vi "SVN Read Method.vi"(6 "Which Method Type":T1, 8 "error in (no error)":errorcluster, 9 "Method version":i32, 10 "Method Name":string) -> (0 "error out":errorcluster, 1 "Valid method":bool, 3 "Method text":string)   [LabVIEW 2012]
uses:
  Which method type.ctl
  ReadWrite.ctl
  Folders.ctl
  Design Server.lvlib
panel:
  out "standard error":string
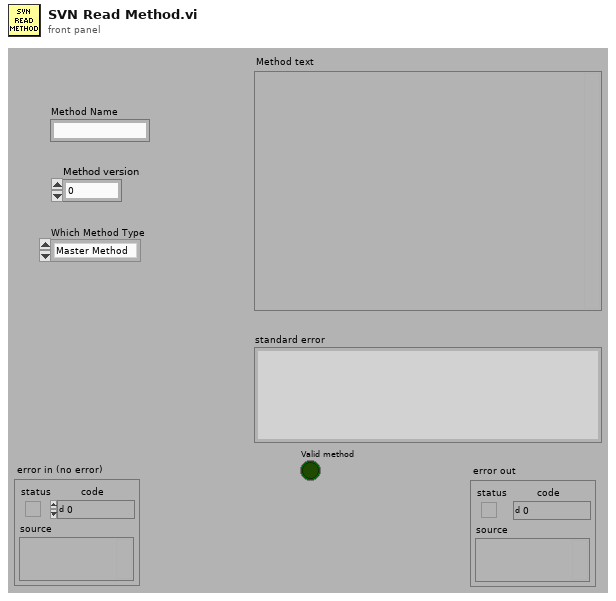
[diagram p1: front panel]
types:
  T1 = typedef "Which method type.ctl" = enum16{"Master Method", "Method"}
  T2 = typedef "Design Server.lvlib/Folders.ctl" = enum16{"MathcadMethods", "RequestedDesigns", "CompletedDesigns", "MathcadCode", "CollabnetSVN.exe"}
  T3 = typedef "ReadWrite.ctl" = enum16{"Read", "Write"}
  T4 = typedef "SVN.ctl" = cluster{"Mathcad Code Repository":string, "Username":string, "Password":string, "Method file names (w extension)":string}
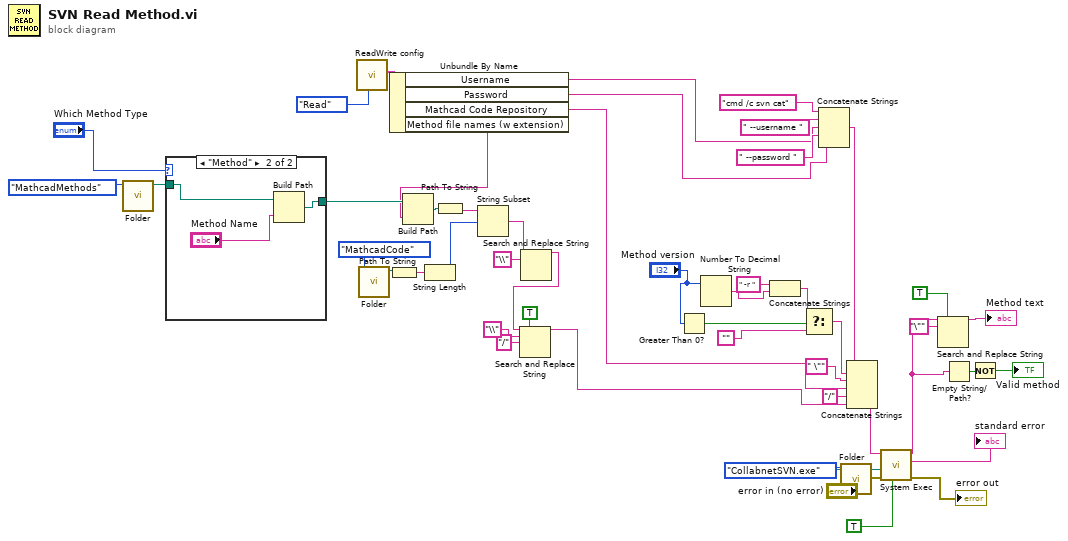
[diagram p0: block diagram]
diagram:
  n1 = call "Folder.vi"("Folders"=Folders."MathcadMethods") -> ("FolderPath"=w22:path)  [unwired: 8 in, 2 out]
  n2 = case shown="\"Method\"" "Which Method Type" {
    tunnel: w22 -> [w50 w53]
    tunnel: [w50 w52] -> w19
    frame "Master Method", Default {
    }
    frame "Method" {
      n3 = Build Path(base path=w53, name or relative path="Method Name") -> (appended path=w52:path)
    }
  }
  n4 = call "ReadWrite config.vi"("Config"=ReadWrite."Read") -> ("SVN"=w37:T4)  [unwired: 7 in, 3 out]
  n5 = call "Folder.vi"("Folders"=Folders."MathcadCode") -> ("FolderPath"=w25:path)  [unwired: 8 in, 2 out]
  n6 = Path To String(path=w25) -> (string=w26:string)
  n7 = Unbundle By Name(w37) -> ("Username"=w34:string, "Password"=w36:string, "Mathcad Code Repository"=w29:string, "Method file names (w extension)"=w1:string)
  n8 = Build Path(base path=w19, name or relative path=w1) -> (appended path=w20:path)
  n9 = String Length(string=w26) -> (length=w21:i32)
  n10 = Path To String(path=w20) -> (string=w17:string)
  n11 = String Subset(string=w17, offset (0)=w21) -> (substring=w18:string)  [unwired: 1 in]
  n12 = Search and Replace String(input string=w18, search string="\\") -> (result string=w12:string)  [unwired: 6 in, 3 out]
  n13 = Search and Replace String(replace all?=TRUE ("replace all? (F)"), input string=w12, search string="\\", replace string="/" ("replace string (\"\")")) -> (result string=w11:string)  [unwired: 4 in, 3 out]
  n14 = Greater Than 0?(x="Method version") -> (x > 0?=w44:bool)
  n15 = Number To Decimal String(number="Method version") -> (decimal integer string=w40:string)  [unwired: 1 in]
  n16 = Concatenate Strings(" -r " ("string"), w40) -> (w42:string)
  n17 = Select(t=w42, s=w44, f="") -> (s? t:f=w39:string)
  n18 = Concatenate Strings("cmd /c svn cat" ("command"), " --username " ("string"), w34, " --password " ("string"), w36) -> (w30:string)
  n19 = call "Folder.vi"("Folders"=Folders."CollabnetSVN.exe") -> ("FolderPath"=w27:path)  [unwired: 8 in, 2 out]
  n20 = Concatenate Strings(w30, w39, " \"" ("string"), w29, "/" ("string"), w11) -> (w15:string)
  n21 = call <vilib>:"System Exec.vi"("run minimized? (F)"=TRUE, "error in (no error)"="error in (no error)", "working directory"=w27, "command line"=w15) -> ("error out"=→"error out":errorcluster, "standard error"=→"standard error":string, "standard output"=w6:string)  [unwired: 4 in, 1 out]
  n22 = Search and Replace String(replace all?=TRUE ("replace all? (F)"), input string=w6, search string="\"") -> (result string=→"Method text":string)  [unwired: 5 in, 3 out]
  n23 = Empty String/Path?(string/path=w6) -> (empty?=w8:bool)
  n24 = Not(x=w8) -> (.not. x?=→"Valid method":bool)
